vi "Set Wash Steps.vi"(8 "error in (no error)":errorcluster, 10 "Wash Steps":T1, 11 "Car Wash Controller in":refnum<class "Car Wash Controller.lvclass">) -> (0 "error out":errorcluster, 3 "Car Wash Controller out":refnum<class "Car Wash Controller.lvclass">)   [LabVIEW 2019, in "Car Wash Controller.lvlib" / "Car Wash Controller.lvclass"]
uses:
  Car Wash Controller.lvclass
  Wash Steps.ctl
  Car Wash Controller.lvclass/Car Wash Controller.ctl
  Sim Wash Display Console/Sim Wash Display Console Messages/Write Wash Step Indicator Msg/Write Wash Step Indicator Msg.lvclass/Write Wash Step Indicator Msg.ctl
  <vilib>/ActorFramework/Message Enqueuer/Message Enqueuer.lvclass/Message Enqueuer.ctl
  <vilib>/ActorFramework/Message Enqueuer/Enqueue.vi
  Sim Wash Display Console/Sim Wash Display Console Messages/Write Wash Step Indicator Msg/Write Wash Step Indicator Msg.lvclass
  C:/Program Files (x86)/National Instruments/LabVIEW 2019/vi.lib/ActorFramework/Message/Message.lvclass
  <vilib>/ActorFramework/Message Priority Queue/Priority Enqueue.vi
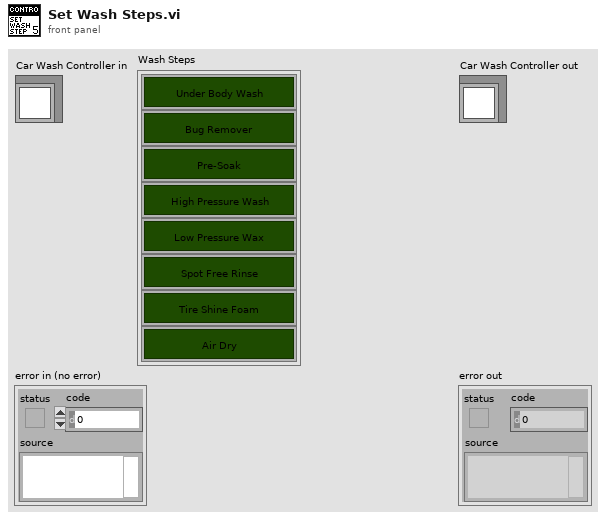
[diagram p1: front panel]
types:
  T1 = typedef "Car Wash Controller.lvlib/Car Wash Controller.lvclass/Wash Steps.ctl" = cluster{"Under Body Wash":bool, "Bug Remover":bool, "Pre-Soak":bool, "High Pressure Wash (Default)":bool, "Low Pressure Wax":bool, "Spot Free Rinse":bool, "Tire Shine Foam":bool, "Air Dry":bool}
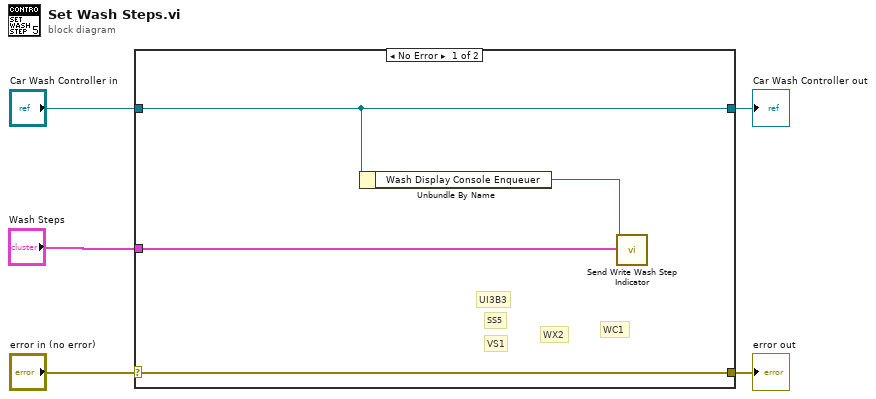
[diagram p0: block diagram]
diagram:
  n1 = case shown="No Error" "error in (no error)" {
    selector: "error in (no error)" -> [w9 w11]
    tunnel: [w9 w11] -> w4
    tunnel: [w8 w10] -> w2
    tunnel: "Car Wash Controller in" -> [w8 w10]
    tunnel: "Wash Steps" -> [w6 _]
    frame No Error {
      # "WC1"
      # "WX2"
      # "VS1"
      # "SS5"
      # "UI3B3"
      n2 = Unbundle By Name(w8) -> ("Wash Display Console Enqueuer"=w7:refnum<class "Message Enqueuer.lvclass">)
      n3 = call "Send Write Wash Step Indicator.vi"("Wash Steps"=w6, "Message Enqueuer"=w7) -> ()  [unwired: 8 in, 2 out]
    }
    frame Error {
    }
  }
  "error out" <- w4
  "Car Wash Controller out" <- w2
